vi "AlazarSetExternalClockLevel.vi"(3 "error in (no error)":errorcluster, 4 "Level (percent)":sgl, 5 "Handle":u64) -> (0 "error out":errorcluster, 1 "Return Code":u32, 2 "Handle":u64)   [LabVIEW 2009]
doc: "Set the external clock comparator level."
uses:
  ATSApi.dll
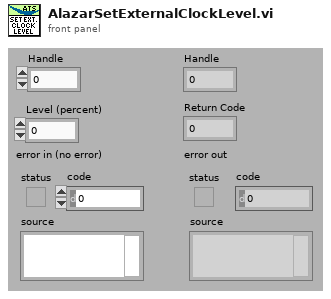
[diagram p1: front panel]
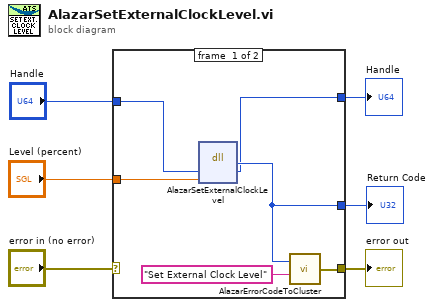
[diagram p0: block diagram]
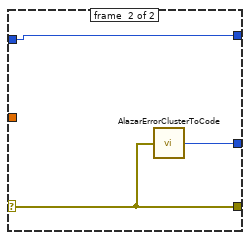
[diagram p2: hidden frame]
diagram:
  n1 = case shown="No Error" "error in (no error)" {
    selector: "error in (no error)" -> [_ w15]
    tunnel: [w9 w15] -> w5
    tunnel: [w11 w14] -> w4
    tunnel: "Handle" -> [w12 w13]
    tunnel: [w8 w13] -> w2
    tunnel: "Level (percent)" -> [w7 _]
    frame #0 {
      n2 = dll-call lib="ATSApi.dll" fn="AlazarSetExternalClockLevel"("handle"=w12, "level_percent"=w7) -> ("return type"=w11:u32, "handle"=w8:u64)  [unwired: 4 in, 2 out]
      n3 = call "AlazarErrorCodeToCluster.vi"("Message"="Set External Clock Level", "Error Code"=w11) -> ("error out"=w9:errorcluster)
    }
    frame #1 {
      n4 = call "AlazarErrorClusterToCode.vi"("error in (no error)"=w15) -> ("Error Code"=w14:u32)
    }
  }
  "Handle" <- w2
  "error out" <- w5
  "Return Code" <- w4
